vi "Get Class Path by Name.vi"(8 "Error in":errorcluster caption="Error in (no error)", 11 "String":string) -> (0 "Error out":errorcluster, 2 "output cluster":T1)   [LabVIEW 2016, in "LV Object Event Registration Node.xnode"]
uses:
  LV Object Event Registration Node.xnode
  LOERN_ClassInfo.ctl
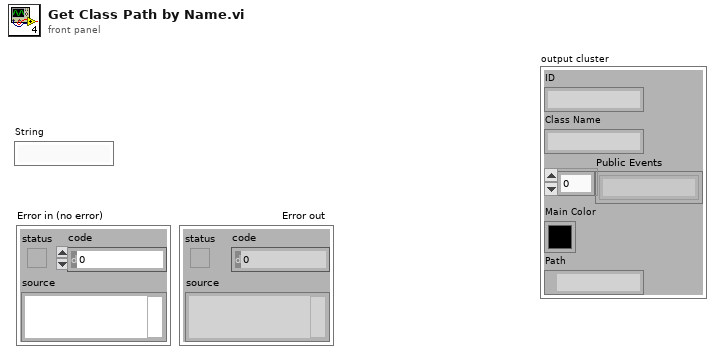
[diagram p1: front panel]
types:
  T1 = typedef "LV Object Event Registration Node.xnode/LOERN_ClassInfo.ctl" = cluster{"ID":string, "Class Name":string, "Public Events":string[], "Main Color":u32, "Path":path}
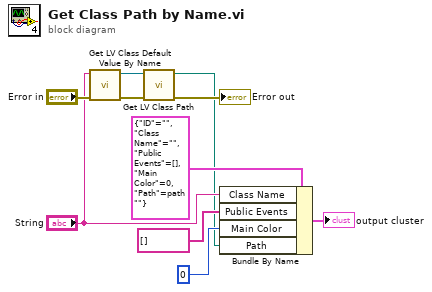
[diagram p0: block diagram]
diagram:
  n1 = call <vilib>:"Get LV Class Default Value By Name.vi"("error in (no error)"="Error in", "class name"="String") -> ("error out"=w10:errorcluster, "object"=w8:refnum<class>)  [unwired: 8 in]
  n2 = call <vilib>:"Get LV Class Path.vi"("error in (no error)"=w10, "object"=w8) -> ("error out"=→"Error out":errorcluster, "class path"=w1:path)  [unwired: 8 in]
  n3 = Bundle By Name(cluster=T1 {"ID"="", "Class Name"="", "Public Events"=[], "Main Color"=0, "Path"=path ""} ("output cluster"), "Class Name"="String", "Public Events"=string[] [], "Main Color"=u32 0, "Path"=w1) -> (→"output cluster":T1)
